vi "LED write.vi"(0 "I2CDevRef":T1={"DevStatus"={"status"=FALSE, "code"=0, "source"=""}, "Controller"=enum."Controller 1", "Device Address"=0, "Handle"=0, "I2C Bus"=enum."Invalid"} {"Device Address" format="%.0x"}, 1 "I2CRegister":u8, 2 "Alliance":T5, 3 "Robot Mode":T4, 4 "Lift Position":u8=35) -> (5 "I2C Byte Output Array":u8[](array[numeric]), 6 "Command":string, 7 "error out":errorcluster)   [LabVIEW 2014]
uses:
  <vilib>/Rock Robotics/WPI/DriverStation/WPI_DriverStationAllianceInfo.ctl
  <vilib>/Rock Robotics/WPI/DriverStation/WPI_DriverStationRobotMode2.ctl
  <vilib>/Rock Robotics/WPI/I2C/WPI_I2CDevRef.ctl
  <vilib>/Rock Robotics/SystemInterfaces/Typedef/FPGA_TypedefDigitalModule.ctl
  <vilib>/Rock Robotics/SystemInterfaces/i2clib/i2c_bus.ctl
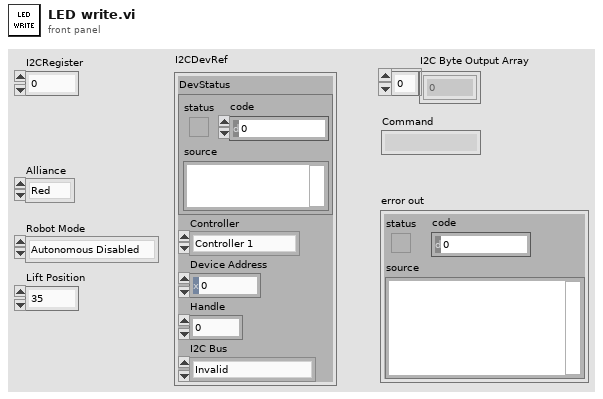
[diagram p1: front panel]
types:
  T1 = typedef "WPI_I2CDevRef.ctl" = cluster{"DevStatus":errorcluster, "Controller":T2, "Device Address":u8, "Handle":i32, "I2C Bus":T3}
  T2 = typedef "FPGA_TypedefDigitalModule.ctl" = enum16{"Controller 1"}
  T3 = typedef "i2c_bus.ctl" = enum16{"I2C On-Board", "I2C MXP", "Invalid"}
  T4 = typedef "WPI_DriverStationRobotMode2.ctl" = enum16{"Autonomous Disabled", "Autonomous Enabled", "Teleop Disabled", "Teleop Enabled", "Disconnected", "Finish", "Test Disabled", "Test Enabled", "Emergency Stopped"}
  T5 = typedef "WPI_DriverStationAllianceInfo.ctl" = enum16{"Red", "Blue", "Invalid"}
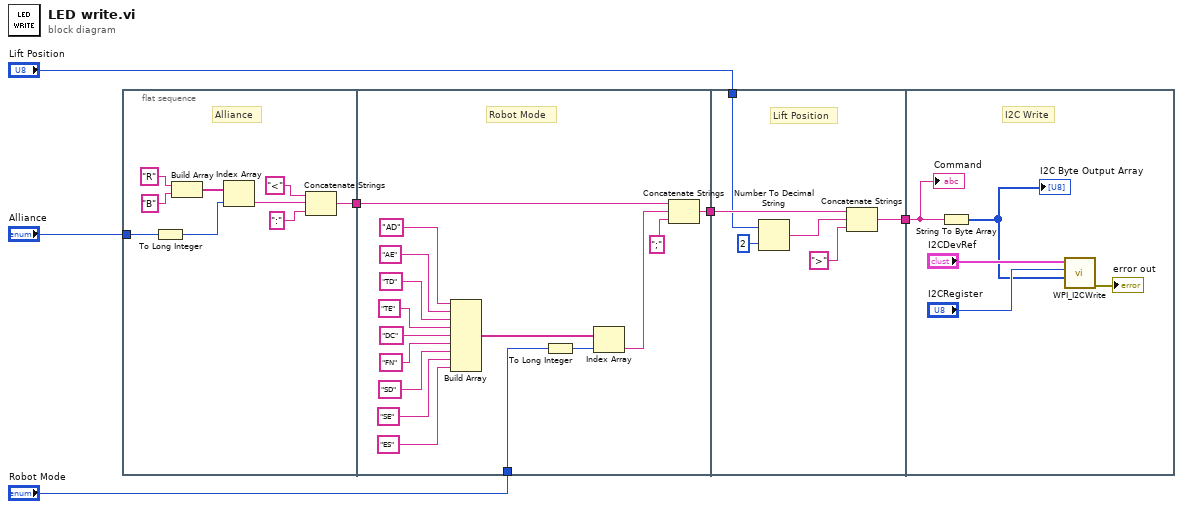
[diagram p0: block diagram]
diagram:
  n1 = flat-sequence {
    tunnel: "Alliance" -> [w8]
    tunnel: [w9] -> w6
    tunnel: w6 -> [w19]
    tunnel: [w18] -> w4
    tunnel: "Robot Mode" -> [w17]
    tunnel: "Lift Position" -> [w32]
    tunnel: w4 -> [w36]
    tunnel: [w33] -> w3
    tunnel: w3 -> [w39]
    frame #0 {
      # "Alliance"
      n2 = To Long Integer(number=w8) -> (32bit integer=w7:i32)
      n3 = Build Array("R", "B") -> (w13:string[])
      n4 = Index Array(array=w13, index=w7) -> (element=w11:string)
      n5 = Concatenate Strings("<", w11, ":") -> (w9:string)
    }
    frame #1 {
      # "Robot Mode"
      n6 = Build Array("AD", "AE", "TD", "TE", "DC", "FN", "SD", "SE", "ES") -> (w22:string[])
      n7 = To Long Integer(number=w17) -> (32bit integer=w16:i32)
      n8 = Index Array(array=w22, index=w16) -> (element=w20:string)
      n9 = Concatenate Strings(w19, w20, ";" ("element")) -> (w18:string)
    }
    frame #2 {
      # "Lift Position"
      n10 = Number To Decimal String(number=w32, width (-)=i16 2) -> (decimal integer string=w35:string)
      n11 = Concatenate Strings(w36, w35, ">") -> (w33:string)
    }
    frame #3 {
      # "I2C Write"
      n12 = String To Byte Array(string=w39) -> (unsigned byte array=w38:u8[])
      "I2C Byte Output Array" <- w38
      n13 = call <vilib>:"WPI_I2CWrite.vi"("I2CDataToSend"=w38, "I2CRegister"="I2CRegister", "I2CDevRef"="I2CDevRef") -> ("error out"=→"error out":errorcluster)  [unwired: 7 in, 1 out]
      "Command" <- w39
    }
  }
